vi "GetRelayCycles.vi"(2 "error in (no error)":errorcluster, 3 "Channel ID":i32=1911 format="%_4g") -> (0 "error out":errorcluster, 1 "N cycles":i32)   [LabVIEW 2009]
doc: "Reads relay cycle count from 34980A"
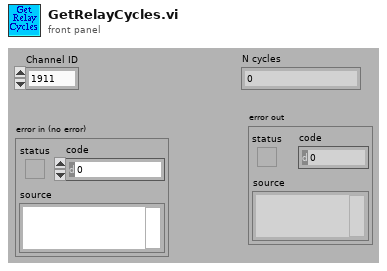
[diagram p1: front panel]
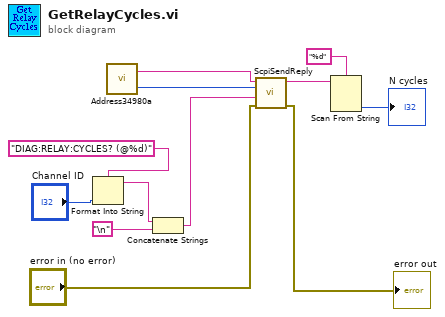
[diagram p0: block diagram]
diagram:
  n1 = Format Into String(format string="DIAG:RELAY:CYCLES? (@%d)", "Channel ID") -> (resulting string=w9:string)  [unwired: 2 in, 1 out]
  n2 = call "Address34980a.vi"() -> ("Port"=w4:i32, "IP address"=w5:string)  [unwired: 2 in]
  n3 = Concatenate Strings(w9, "\n") -> (w8:string)
  n4 = call "ScpiSendReply.vi"("error in (no error)"="error in (no error)", "Command"=w8, "TCP port"=w4, "IP Address"=w5) -> ("Error out"=→"error out":errorcluster, "Reply"=w1:string)  [unwired: 5 in]
  n5 = Scan From String(format string="%d", input string=w1) -> (output 1=→"N cycles":i32)  [unwired: 3 in, 3 out]
